vi "Unlock Data.vi"(8 "error in (no error)":errorcluster caption="错误输入（无错误）", 11 "asicHandle":i32) -> (0 "error out":errorcluster caption="错误输出", 3 "function return":i32)   [LabVIEW 2020]
doc: "extern int __stdcall APSxUnlockData (int asicHandle );"
uses:
  APSx.dll/APSx.dll
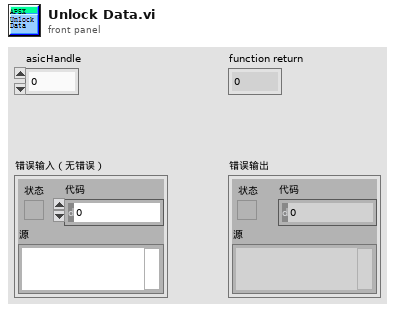
[diagram p1: front panel]
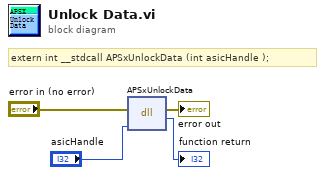
[diagram p0: block diagram]
diagram:
  # "extern int __stdcall APSxUnlockData (int asicHandle );"
  n1 = dll-call lib="PTH2Mabs D程序临时修改280传感器对中台SourcesAPSx.dllAPSx.*" fn="APSxUnlockData"(error in="error in (no error)", "asicHandle"="asicHandle") -> (error out=→"error out":errorcluster, →"function return":i32)  [unwired: 3 in, 1 out]
